vi "ObjectHandler.GetRefWithoutAdd.vi"(8 "error in (no error)":errorcluster, 10 "data":T1={"Name"="", "ObjectWType"={"ObjectType"=enum."ObjectHandler", "Object"=variant(refnum<data-value> refnum)}, "Caller"=""}, 11 "ObjectHandler in":refnum<class "ObjectHandler.lvclass">) -> (0 "error out":errorcluster, 3 "ObjectHandler out":refnum<class "ObjectHandler.lvclass">)   [LabVIEW 2016, in "ObjectHandler.lvclass"]
uses:
  ObjectHandler.lvclass
  ObjectHandler.ObjectMessageWCaller.ctl
  ObjectHandler.ObjectWType.ctl
  ObjectHandler.ObjectType.ctl
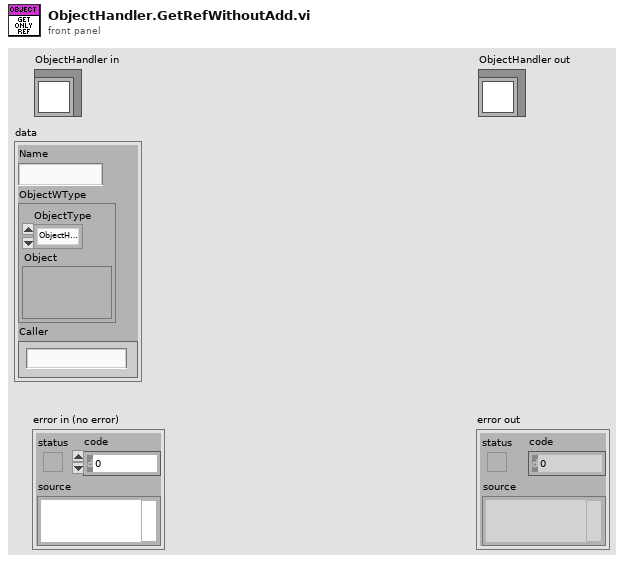
[diagram p1: front panel]
types:
  T1 = typedef "ObjectHandler.lvclass/ObjectHandler.ObjectMessageWCaller.ctl" = cluster{"Name":string, "ObjectWType":T2, "Caller":string}
  T2 = typedef "ObjectHandler.lvclass/ObjectHandler.ObjectWType.ctl" = cluster{"ObjectType":T3, "Object":variant}
  T3 = typedef "ObjectHandler.lvclass/ObjectHandler.ObjectType.ctl" = enum16{"undefined", "ObjectHandler", "ViHandler", "ErrorHandler", "CentralStorage", "Hausmodell", "Sondenmodell", "Wärmepumpe", "Umgebung"}
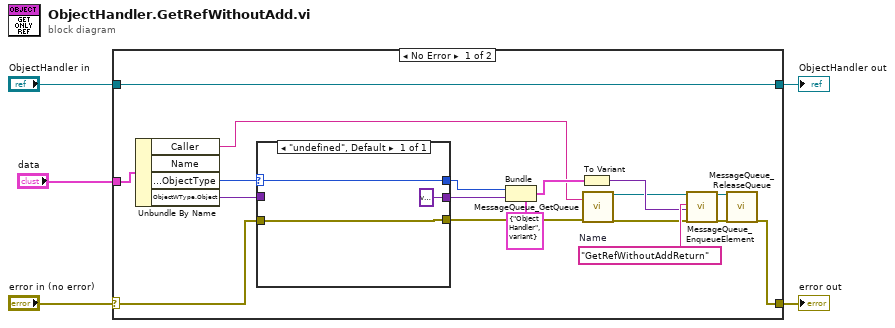
[diagram p0: block diagram]
diagram:
  n1 = case shown="No Error" "error in (no error)" {
    selector: "error in (no error)" -> [w18 w27]
    tunnel: [w7 w27] -> w4
    tunnel: [w16 w28] -> w2
    tunnel: "ObjectHandler in" -> [w16 w28]
    tunnel: "data" -> [w23 _]
    frame No Error {
      w15 = "GetRefWithoutAddReturn"  # Name
      n2 = Unbundle By Name(w23) -> ("Caller"=w9:string, "ObjectWType.ObjectType"=w21:T3, "ObjectWType.Object"=w19:variant)  [unwired: 1 out]
      n3 = case shown="\"undefined\", Default" w21 {
        selector: w21 -> [w26]
        tunnel: [w26] -> w20
        tunnel: w19 -> [_]
        tunnel: w18 -> [w24]
        tunnel: [w24] -> w8
        tunnel: [variant ("Variant")] -> w17
        frame "undefined", Default {
        }
      }
      n4 = Bundle(cluster=T2 {"ObjectType"=enum."ObjectHandler", "Object"=variant} ("ObjectWType"), "ObjectType"=w20, "Object"=w17) -> (w10:T2)
      n5 = To Variant(anything=w10) -> (Variant=w14:variant)
      n6 = call "MessageQueue_GetQueue.vi"("Name"=w9, "ErrorIn"=w8) -> ("QueueOut"=w11:refnum<queue>, "ErrorOut"=w6:errorcluster)  [unwired: 15 in, 1 out]
      n7 = call "MessageQueue_EnqueueElement.vi"("QueueIn"=w11, "Message"=w15, "Data"=w14, "ErrorIn"=w6) -> ("QueueOut"=w13:refnum<queue>, "ErrorOut"=w12:errorcluster)  [unwired: 14 in]
      n8 = call "MessageQueue_ReleaseQueue.vi"("QueueIn"=w13, "ErrorIn"=w12) -> ("ErrorOut"=w7:errorcluster)  [unwired: 15 in, 2 out]
    }
    frame Error {
    }
  }
  "error out" <- w4
  "ObjectHandler out" <- w2
